vi "PV ASM340 Special.vi"(7 "Adress of unit":u16=1 min=1 max=999 step=1, 8 "error in (no error)":errorcluster, 9 "PV ASM340 Special - Cluster":T1={"Parameter"=0, "Parameter\nread only<->describe"=FALSE, "Anodenpotential Mass 2"=905, "Anodenpotential Mass 3"=610, "Anodenpotential Mass 4"=465, "Filament"=0} {"Filament" items=["Emission off", "Filament 1, emission on", "Filament 2, emission on"]; "Anodenpotential Mass 4" min=390 max=520 step=1; "Anodenpotential Mass 3" min=510 max=610 step=1; "Anodenpotential Mass 2" min=785 max=995 step=1; "Parameter" items=[" Anodenpotential Mass 2 [V] (631)", " Anodenpotential Mass 3 [V] (632)", " Anodenpotential Mass 4 [V] (633)", " Filament (645)"]}, 11 "VISA session":refnum<visa-resource-name>) -> (0 "error out":errorcluster, 2 "response (data)":string, 3 "dup VISA session":refnum<visa-resource-name>)   [LabVIEW 2021, in "Pfeiffer Vacuum.lvlib"]
doc: "There are 4 parameters available, only one of which can be enabled at a time. \n\n0 - Anodenpotential Mass 2 [V] - Para 631\n1 - Anodenpotential Mass 3 [V] - Para 632\n2 - Anodenpotential Mass 4 [V] - Para 633\n3 - Filament - Para 645\n\nNote: Any settings for an parameter that is not selected will be ignored. If a value is out of range, it will be changed to either the upper or the lower limit of the range."
uses:
  <instrlib>/Pfeiffer Vacuum/Pfeiffer Vacuum.lvlib
  <instrlib>/Pfeiffer Vacuum/Public/LeakDetector ASM340/PV ASM340 Special - Cluster.ctl
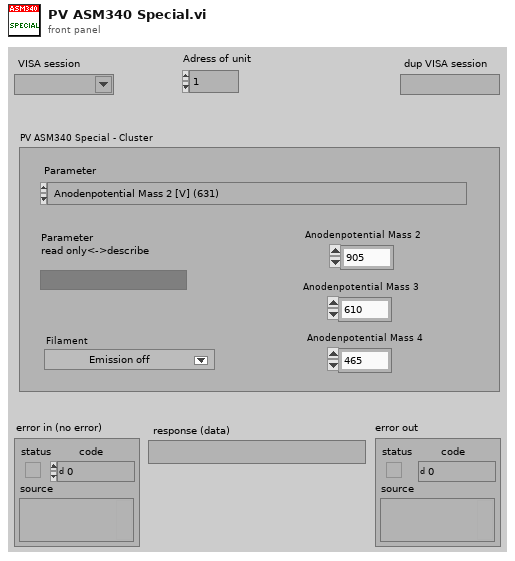
[diagram p1: front panel]
types:
  T1 = typedef "Pfeiffer Vacuum.lvlib/PV ASM340 Special - Cluster.ctl" = cluster{"Parameter":u16, "Parameter\nread only<->describe":bool, "Anodenpotential Mass 2":u16, "Anodenpotential Mass 3":u16, "Anodenpotential Mass 4":u16, "Filament":u16}
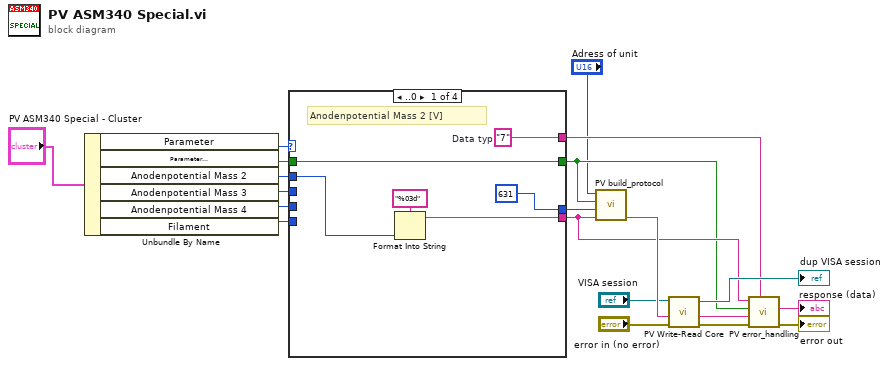
[diagram p0: block diagram]
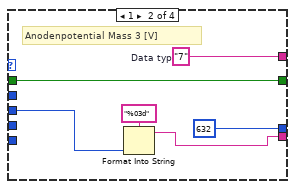
[diagram p2: hidden frame]
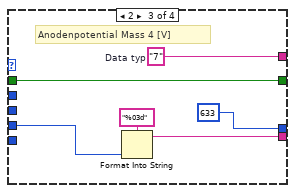
[diagram p3: hidden frame]
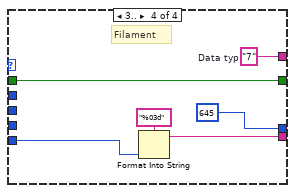
[diagram p4: hidden frame]
diagram:
  n1 = Unbundle By Name("PV ASM340 Special - Cluster") -> ("Parameter"=w8:u16, "Parameter\nread only<->describe"=w19:bool, "Anodenpotential Mass 2"=w9:u16, "Anodenpotential Mass 3"=w6:u16, "Anodenpotential Mass 4"=w5:u16, "Filament"=w4:u16)
  n2 = case shown="..0" w8 {
    tunnel: [u16 631 ("Parameter-number") u16 632 ("Parameter-number") u16 633 ("Parameter-number") u16 645 ("Parameter-number")] -> w20
    tunnel: [w21 w27 w33 w40] -> w14
    tunnel: [w24 w30 w36 w42] -> w12
    tunnel: w19 -> [w24 w30 w36 w42]
    tunnel: [w26 w32 w38 w44] -> w13
    tunnel: w9 -> [w22 _ _ _]
    tunnel: w6 -> [_ w28 _ _]
    tunnel: w5 -> [_ _ w34 _]
    tunnel: w4 -> [_ _ _ w39]
    frame ..0 {
      w26 = "7"  # Data typ
      # "Anodenpotential Mass 2 [V]"
      n3 = Format Into String(format string="%03d" ("Format-String"), w22) -> (resulting string=w21:string)  [unwired: 2 in, 1 out]
    }
    frame 1 {
      w32 = "7"  # Data typ
      # "Anodenpotential Mass 3 [V]"
      n4 = Format Into String(format string="%03d" ("Format-String"), w28) -> (resulting string=w27:string)  [unwired: 2 in, 1 out]
    }
    frame 2 {
      w38 = "7"  # Data typ
      # "Anodenpotential Mass 4 [V]"
      n5 = Format Into String(format string="%03d" ("Format-String"), w34) -> (resulting string=w33:string)  [unwired: 2 in, 1 out]
    }
    frame 3.. {
      w44 = "7"  # Data typ
      # "Filament"
      n6 = Format Into String(format string="%03d" ("Format-String"), w39) -> (resulting string=w40:string)  [unwired: 2 in, 1 out]
    }
  }
  n7 = call <instrlib>:"PV build_protocol.vi"("Data"=w14, "Parameter-number"=w20, "parameter\nread<->describe"=w12, "Adress"="Adress of unit") -> ("output"=w18:string)  [unwired: 3 in]
  n8 = call <instrlib>:"PV Write-Read Core.vi"("error in"="error in (no error)", "Write data in"=w18, "VISA session"="VISA session") -> ("error out"=w16:errorcluster, "response (data) out"=w17:string, "dup VISA session"=→"dup VISA session":refnum<visa-resource-name>)  [unwired: 2 in]
  n9 = call <instrlib>:"PV error_handling.vi"("Data Typ in"=w13, "error in"=w16, "response (data) in"=w17, "Parameter\nread only<->describe"=w12, "data in"=w14) -> ("error out"=→"error out":errorcluster, "Data out"=→"response (data)":string)  [unwired: 4 in, 1 out]
